vi "State_Machine.vi"(8 "error in (no error)":errorcluster caption="entrée d'erreur (pas d'erreur)", 11 "Delay en entrée":refnum<class "P2056_Provisionning.lvclass">) -> (0 "error out":errorcluster caption="sortie d'erreur", 2 "Json_String":string, 3 "Delay en sortie":refnum<class "P2056_Provisionning.lvclass">)   [LabVIEW 2020, in "Library Test.lvlib" / "P2056_Provisionning.lvclass"]
uses:
  P2056_Provisionning.lvclass
  C:/Users/ngarcin/OneDrive - Altyor/Standard TB/Suite TB45/Class/Test/Test (Default)/Test (Default).lvclass
  Commun VI/TypeDef/Variable Printable.ctl
  Read CSV File/Class File (Default)/Class File (Default).lvclass
  JSON API/JSON Value/Set from JSON string.vi
  JSON API/Variant JSON/Variant to JSON.vi
  JSON API/JSON Value/Get Item by name array.vi
  JSON API/JSON Value/JSON Value.lvclass
  JSON API/Variant JSON/Variant JSON.lvlib
  JSON API/Get Polymorphic/JSON GetSet.lvlib
  Commun VI/Library Commun.lvlib
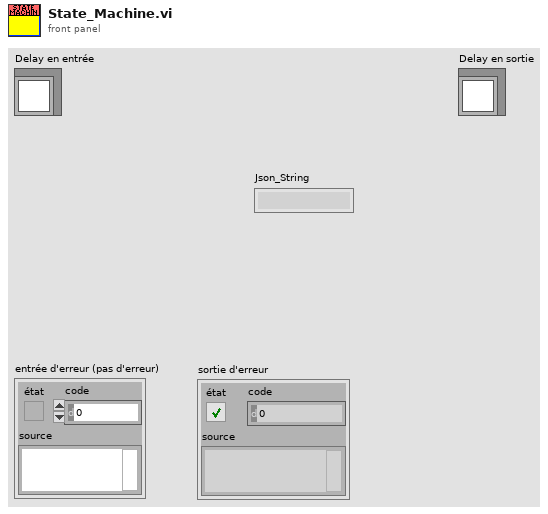
[diagram p1: front panel]
types:
  T1 = typedef "Variable Printable.ctl" = string
  T2 = cluster{"deviceID":string, "serialNumber":string, "popCode":string, "IMEI":string, "ICCID":string, "mfgDate":string}
  T3 = cluster{"iotInterfaces":cluster{"deviceID":string, "serialNumber":string, "popCode":string, "IMEI":string, "ICCID":string, "mfgDate":string}[]}
  T4 = cluster{"Path file Json":path, "Server":string, "Profile":string}
  T5 = enum16{"Get Variable", "Get All Variables", "Set Variable", "Delete Variable", "Delete All Variable"}
  T6 = cluster{"deviceID":string, "serialNumber":string, "popCode":string, "IMEI":string, "ICCID":string, "mfgDate":string}[]
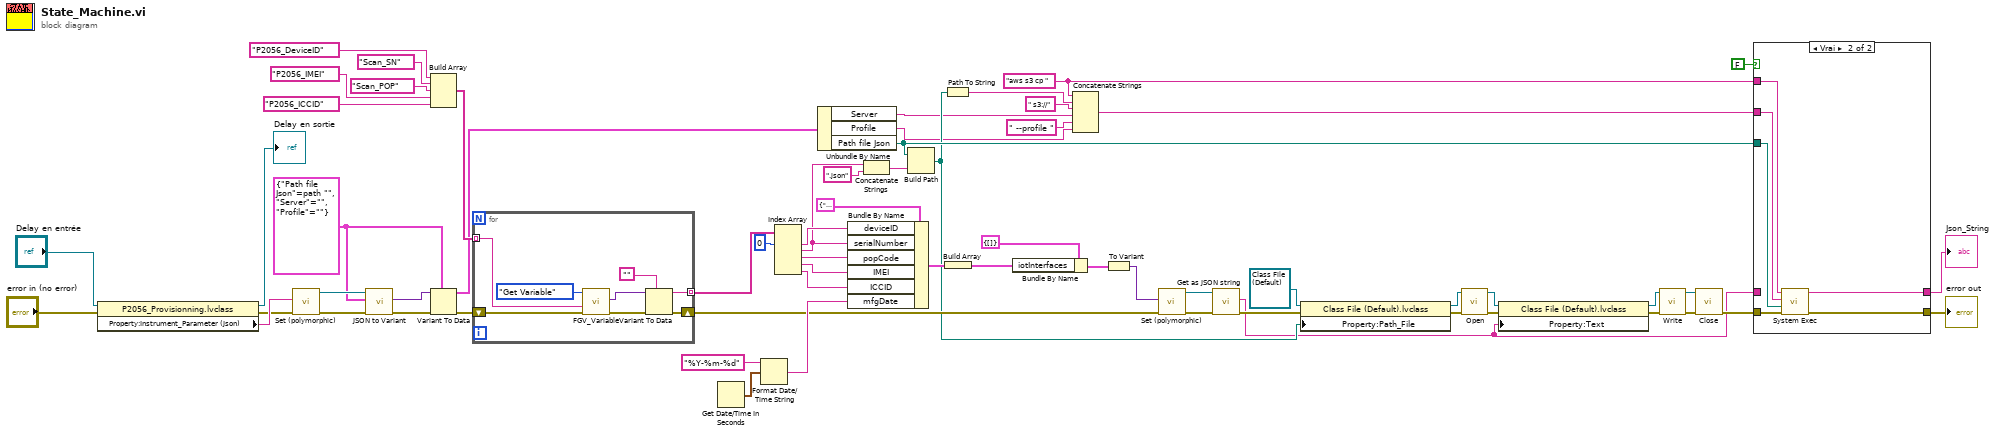
[diagram p0: block diagram]
diagram:
  w10 = "aws s3 cp " ("command line")
  w55 = T4 {"Path file Json"=path "", "Server"="", "Profile"=""}
  n1 = property class="P2056_Provisionning.lvclass"(reference="Delay en entrée", error in="error in (no error)") -> (reference out=→"Delay en sortie":refnum<class "P2056_Provisionning.lvclass">, error out=w56:errorcluster, "Property:Instrument_Parameter (Json)"=w58:string)
  n2 = call-poly "Set (polymorphic).vi"("error in (no error)"=w56, "JSON stream"=w58) -> ("error out"=w60:errorcluster, "JSON Value out"=w62:refnum<class "JSON Value.lvclass">)  [unwired: 7 in, 1 out]
  n3 = call "JSON to Variant.vi"("error in (no error)"=w60, "Variant (Data Type)"=w55, "JSON Value"=w62) -> ("error out"=w61:errorcluster, "Variant out"=w59:variant)  [unwired: 7 in]
  n4 = Build Array(T1 "P2056_DeviceID" ("Variable"), T1 "Scan_SN" ("Variable"), T1 "Scan_POP" ("Variable"), T1 "P2056_IMEI" ("Variable"), T1 "P2056_ICCID" ("Variable")) -> (w46:T1[])
  n5 = Variant To Data(error in=w61, type=w55, Variant=w59) -> (data=w18:T4, error out=w54:errorcluster)
  n6 = for {
    tunnel: w46 -> [w66] mode=indexing
    shift-right: [w65] -> w28
    shift-left: w54 -> [w71]
    tunnel: [w64] -> w44 mode=indexing
    n7 = call "FGV_Variable.vi"("error in (no error)"=w71, "Variable"=w66, "Function"=T5."Get Variable") -> ("error out"=w70:errorcluster, "Data Out"=w68:variant)  [unwired: 6 in, 1 out]
    n8 = Variant To Data(error in=w70, type="", Variant=w68) -> (data=w64:string, error out=w65:errorcluster)
  }
  n9 = Get Date/Time In Seconds() -> (seconds since 1Jan1904=w36:timestamp)
  n10 = Format Date/Time String(time format string (%c)="%Y-%m-%d" ("chaîne de format de l'heure (%c)"), seconds (now)=w36) -> (date/time string=w34:string)  [unwired: 1 in]
  n11 = Index Array(array=w44, index #1=0 ("indice")) -> (element #1=w42:string, element #2=w17:string, element #3=w41:string, element #4=w39:string, element #5=w37:string)  [unwired: 4 in]
  n12 = Unbundle By Name(w18) -> ("Server"=w6:string, "Profile"=w3:string, "Path file Json"=w12:path)
  n13 = Bundle By Name(cluster=T2 {"deviceID"="", "serialNumber"="", "popCode"="", "IMEI"="", "ICCID"="", "mfgDate"=""}, "deviceID"=w42, "serialNumber"=w17, "popCode"=w41, "IMEI"=w39, "ICCID"=w37, "mfgDate"=w34) -> (w51:T2)
  n14 = Concatenate Strings(w17, ".json" ("chaîne")) -> (w15:string)
  n15 = Build Path(base path=w12, name or relative path=w15) -> (appended path=w9:path)
  n16 = Path To String(path=w9) -> (string=w8:string)
  n17 = Build Array(w51) -> (w50:T6)
  n18 = Bundle By Name(cluster=T3 {"iotInterfaces"=[]}, "iotInterfaces"=w50) -> (w29:T3)
  n19 = Concatenate Strings(w10, w8, " s3://" ("chaîne"), w6, " --profile " ("chaîne"), w3) -> (w4:string)
  n20 = To Variant(anything=w29) -> (Variant=w32:variant)
  n21 = call-poly "Set (polymorphic).vi"("error in (no error)"=w28, "Variant"=w32) -> ("error out"=w30:errorcluster, "JSON Value out"=w31:refnum<class "JSON Value.lvclass">)  [unwired: 8 in]
  n22 = call "Get as JSON string.vi"("error in (no error)"=w30, "JSON Value in"=w31) -> ("error out"=w14:errorcluster, "<JSON>"=w1:string)  [unwired: 8 in]
  n23 = property class="Class File (Default).lvclass"(reference=refnum<class "Class File (Default).lvclass"> refnum ("Library File.lvlib:Class File (Default).lvclass"), error in=w14, "Property:Path_File"=w9) -> (reference out=w27:refnum<class "Class File (Default).lvclass">, error out=w26:errorcluster)
  n24 = call-dynamic "Open.vi"("error in (no error)"=w26, "Class CSV_File (Default) en entrée"=w27) -> ("error out"=w24:errorcluster, "Class CSV_File (Default) en sortie"=w23:refnum<class "Class File (Default).lvclass">)  [unwired: 8 in]
  n25 = property class="Class File (Default).lvclass"(reference=w23, error in=w24, "Property:Text"=w1) -> (reference out=w22:refnum<class "Class File (Default).lvclass">, error out=w20:errorcluster)
  n26 = call-dynamic "Write.vi"("error in (no error)"=w20, "Class CSV_File (Default) en entrée"=w22) -> ("error out"=w19:errorcluster, "Class CSV_File (Default) en sortie"=w21:refnum<class "Class File (Default).lvclass">)  [unwired: 8 in]
  n27 = call-dynamic "Close.vi"("error in (no error)"=w19, "Class CSV_File (Default) en entrée"=w21) -> ("error out"=w13:errorcluster)  [unwired: 8 in, 1 out]
  n28 = case shown="Vrai" FALSE {
    tunnel: [w73 w79] -> w33
    tunnel: w13 -> [w73 w78]
    tunnel: w12 -> [_ w77]
    tunnel: [w72 w76] -> w11
    tunnel: w10 -> [_ w75]
    tunnel: w4 -> [_ w74]
    tunnel: w1 -> [w72 _]
    frame False {
    }
    frame True {
      n29 = call <vilib>:"System Exec.vi"("error in (no error)"=w78, "working directory"=w77, "standard input"=w74, "command line"=w75) -> ("error out"=w79:errorcluster, "standard output"=w76:string)  [unwired: 4 in, 2 out]
    }
  }
  "Json_String" <- w11
  "error out" <- w33
